vi "Next Step.vi"(8 "error in (no error)":errorcluster, 11 "Magna Power Scan in":refnum<class "Magna Power Scan.lvclass">) -> (0 "error out":errorcluster, 1 "Current Step":u32, 2 "Current Position":dbl, 3 "Magna Power Scan out":refnum<class "Magna Power Scan.lvclass">)   [LabVIEW 2012, in "Magna Power Scan.lvclass"]
doc: "(Dynamic) Move to the next preconfigured step of this Scanner, and return the current position (actual, not intended) of this Scanner. Increment the step counter by one."
uses:
  Magna Power Scan.lvclass
  Instruments/Magna-Power Power Supply/Magna Power.lvclass
  Scanner/Scanner.lvclass
  Magna Power Scan.lvclass/Magna Power Scan.ctl
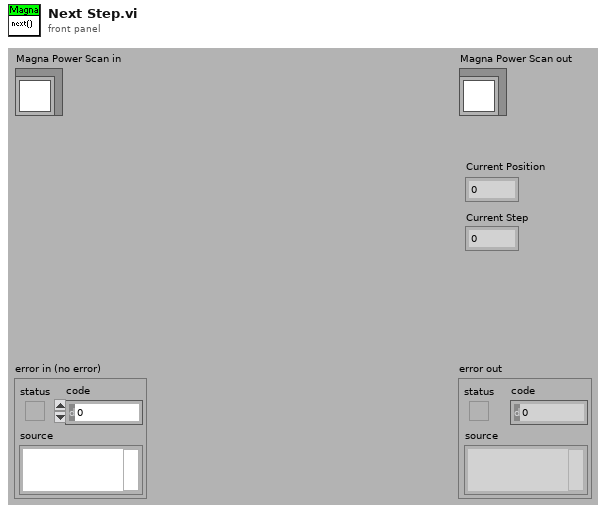
[diagram p1: front panel]
types:
  T1 = typedef "Scanner.lvclass/Range.ctl" = cluster{"xi":dbl, "xf":dbl, "dx":dbl, "Return to...?":bool, "Return to":dbl}
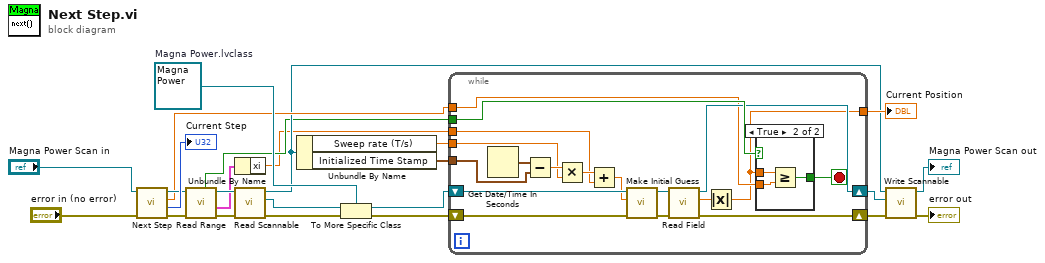
[diagram p0: block diagram]
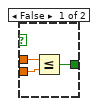
[diagram p2: hidden frame]
diagram:
  w19 = refnum<class "Magna Power.lvclass"> refnum  # Magna Power.lvclass
  n1 = call-parent "Next Step.vi"("error in (no error)"="error in (no error)", "Scanner in"="Magna Power Scan in") -> ("error out"=w18:errorcluster, "Current Step"=→"Current Step":u32, "Current Position"=w9:dbl, "Scanner out"=w16:refnum<class "Magna Power Scan.lvclass">)  [unwired: 6 in]
  n2 = call-dynamic "Read Range.vi"("error in (no error)"=w18, "Scanner.lvclass in"=w16) -> ("error out"=w17:errorcluster, "Range"=w14:T1, "Scanner.lvclass out"=w15:refnum<class "Magna Power Scan.lvclass">, "Scanning Up?"=w2:bool)  [unwired: 4 in, 2 out]
  n3 = Unbundle By Name(w14) -> ("xi"=w1:dbl)
  n4 = call-dynamic "Read Scannable.vi"("error in (no error)"=w17, "Scanner.lvclass in"=w15) -> ("error out"=w21:errorcluster, "Scannable.lvclass"=w20:refnum<class "Scannable.lvclass">, "Scanner.lvclass out"=w3:refnum<class "Magna Power Scan.lvclass">)  [unwired: 7 in]
  n5 = Unbundle By Name(w3) -> ("Sweep rate (T/s)"=w12:dbl, "Initialized Time Stamp"=w13:timestamp)
  n6 = To More Specific Class(target class=w19, reference=w20, error in=w21) -> (specific class reference=w10:refnum<class "Magna Power.lvclass">, error out=w11:errorcluster)
  n7 = while {
    tunnel: w13 -> [w41]
    tunnel: w12 -> [w39]
    shift-right: [w30] -> w7
    shift-left: w11 -> [w37]
    shift-right: [w31] -> w6
    shift-left: w10 -> [w36]
    tunnel: w2 -> [w32]
    tunnel: w9 -> [w29]
    tunnel: [w25] -> w8
    tunnel: w1 -> [w27]
    stop <- w28 stop-if-true
    n8 = Get Date/Time In Seconds() -> (seconds since 1Jan1904=w42:timestamp)
    n9 = Subtract(x=w42, y=w41) -> (x-y=w40:dbl)
    n10 = Multiply(x=w40, y=w39) -> (x*y=w38:dbl)
    n11 = Add(x=w38, y=w27) -> (x+y=w35:dbl)
    n12 = call "Make Initial Guess.vi"("error in (no error)"=w37, "Desired Field"=w35, "Magna Power in"=w36) -> ("error out"=w34:errorcluster, "Magna Power out"=w33:refnum<class "Magna Power.lvclass">)  [unwired: 6 in, 1 out]
    n13 = call "Read Field.vi"("error in (no error)"=w34, "Magna Power in"=w33) -> ("error out"=w30:errorcluster, "Field (T)"=w26:dbl, "Magna Power out"=w31:refnum<class "Magna Power.lvclass">)  [unwired: 7 in]
    n14 = Absolute Value(x=w26) -> (abs(x)=w25:dbl)
    n15 = case shown="True" w32 {
      tunnel: w25 -> [w45 w46]
      tunnel: w29 -> [w44 w48]
      tunnel: [w43 w47] -> w28
      frame False {
        n16 = Less Or Equal?(x=w45, y=w44) -> (x <= y?=w43:bool)
      }
      frame True {
        n17 = Greater Or Equal?(x=w46, y=w48) -> (x >= y?=w47:bool)
      }
    }
  }
  "Current Position" <- w8
  n18 = call-dynamic "Write Scannable.vi"("error in (no error)"=w7, "Scannable.lvclass"=w6, "Scanner.lvclass in"=w3) -> ("error out"=→"error out":errorcluster, "Scanner.lvclass out"=→"Magna Power Scan out":refnum<class "Magna Power Scan.lvclass">)  [unwired: 7 in]
